vi "Create Sensor Object.vi"(8 "error in (no error)":errorcluster caption="错误输入（无错误）", 9 "sensorHandle":i32, 10 "sensorName":string, 11 "pgiType":i32) -> (0 "error out":errorcluster caption="错误输出", 1 "sensorHandle out":i32, 2 "sensorName out":string, 3 "function return":i32)   [LabVIEW 2020]
doc: "extern int __stdcall APSxCreateSensorObject (IN int pgiType, IN char * sensorName, OUT int * sensorHandle);"
uses:
  APSx.dll/APSx.dll
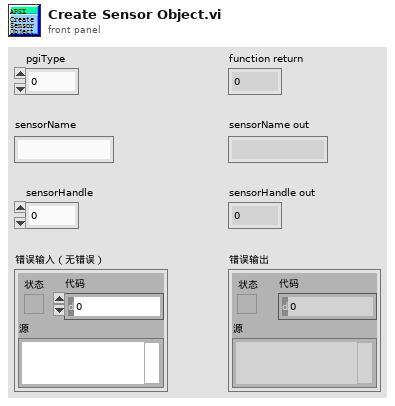
[diagram p1: front panel]
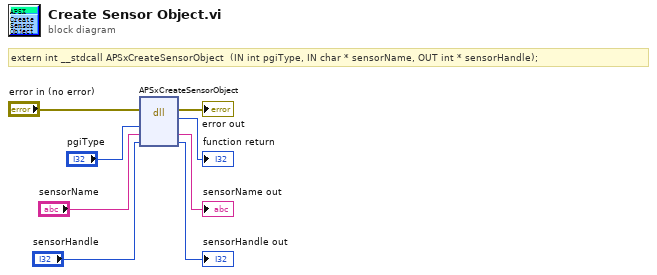
[diagram p0: block diagram]
diagram:
  # "extern int __stdcall APSxCreateSensorObject  (IN int pgiType, IN char * sensorName, OUT int * sensorHandle);"
  n1 = dll-call lib="PTH2iabs CUsersFengDesktop传感器对中台传感器对中台labviewSourcesAPSx.dllAPSx.dll" fn="APSxCreateSensorObject"(error in="error in (no error)", "pgiType"="pgiType", "sensorName"="sensorName", "sensorHandle"="sensorHandle") -> (error out=→"error out":errorcluster, "返回类型"=→"function return":i32, "sensorName"=→"sensorName out":string, "sensorHandle"=→"sensorHandle out":i32)  [unwired: 3 in, 1 out]
